vi "Button selection(SubVI).vi"(11 "button info":T1) -> (3 "Cluster":T2)   [LabVIEW 2014]
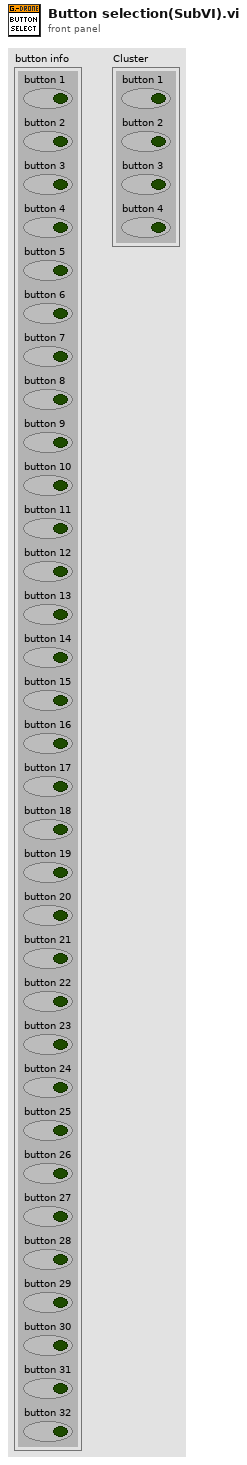
[diagram p1: front panel]
types:
  T1 = cluster{"button 1":bool, "button 2":bool, "button 3":bool, "button 4":bool, "button 5":bool, "button 6":bool, "button 7":bool, "button 8":bool, "button 9":bool, "button 10":bool, "button 11":bool, "button 12":bool, "button 13":bool, "button 14":bool, "button 15":bool, "button 16":bool, "button 17":bool, "button 18":bool, "button 19":bool, "button 20":bool, "button 21":bool, "button 22":bool, "button 23":bool, "button 24":bool, "button 25":bool, "button 26":bool, "button 27":bool, "button 28":bool, "button 29":bool, "button 30":bool, "button 31":bool, "button 32":bool}
  T2 = cluster{"button 1":bool, "button 2":bool, "button 3":bool, "button 4":bool}
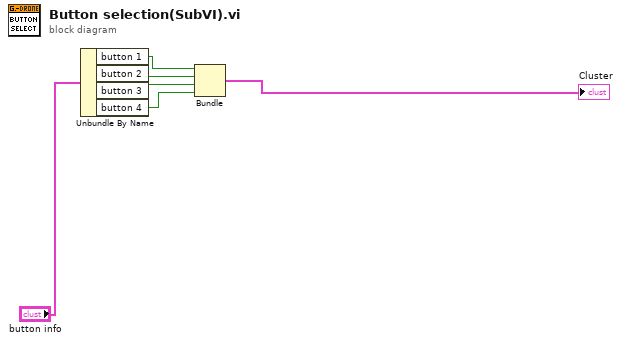
[diagram p0: block diagram]
diagram:
  n1 = Unbundle By Name("button info") -> ("button 1"=w2:bool, "button 2"=w3:bool, "button 3"=w4:bool, "button 4"=w5:bool)
  n2 = Bundle("button 1"=w2, "button 2"=w3, "button 3"=w4, "button 4"=w5) -> (→"Cluster":T2)  [unwired: 1 in]
